vi "Do Draw.vi"(9 "color":u32(colorbox), 10 "picture in":picture, 11 "Reset Message":refnum<class "Reset Message.lvclass">) -> (2 "picture out":picture)   [LabVIEW 2023, in "Draw Messages.lvlib" / "Reset Message.lvclass"]
doc: "Draw whatever the message needs to draw into the picture."
uses:
  Reset Message.lvclass
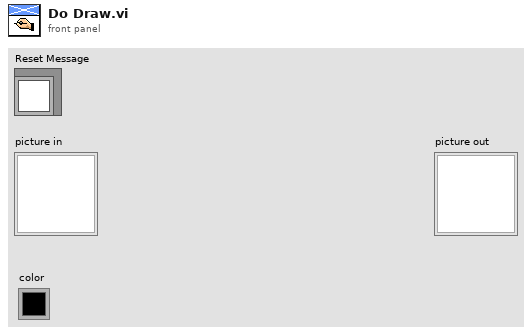
[diagram p1: front panel]
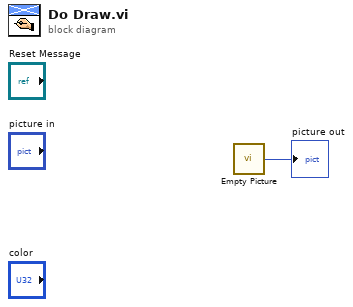
[diagram p0: block diagram]
diagram:
  n1 = call "Empty Picture"() -> ("empty picture"=→"picture out":picture)
